vi "Decode data format.vi"(11 "Generic packet":T3) -> (1 "XAM Data Packet":T1, 2 "IDRA Data Packet":T2, 3 "Telemetria.Data format":enum16{"IDRA data", "XAM data"}(ring))   [LabVIEW 2015, in "Acquisition.lvlib"]
uses:
  Acquisition.lvlib
  Generic data packet.ctl
  My Graphs/Gps Map Graph coordinates.ctl
  IDRA Data Packet.ctl
  XAM Data Packet.ctl
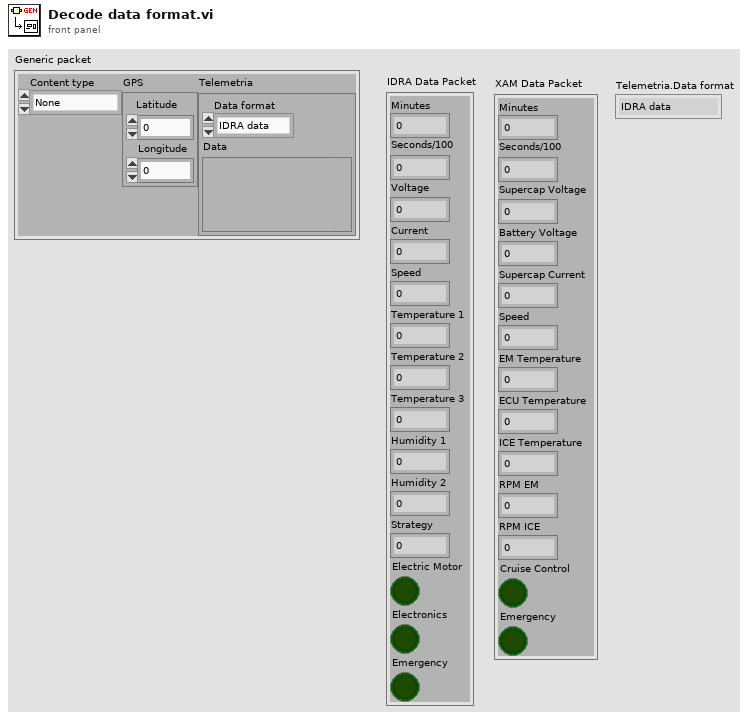
[diagram p1: front panel]
types:
  T1 = typedef "Acquisition.lvlib/XAM Data Packet.ctl" = cluster{"Minutes":u16, "Seconds/100":u16, "Supercap Voltage":sgl, "Battery Voltage":sgl, "Supercap Current":sgl, "Speed":sgl, "EM Temperature":sgl, "ECU Temperature":sgl, "ICE Temperature":sgl, "RPM EM":u16, "RPM ICE":u16, "Cruise Control":bool, "Emergency":bool}
  T2 = typedef "Acquisition.lvlib/IDRA Data Packet.ctl" = cluster{"Minutes":u16, "Seconds/100":u16, "Voltage":sgl, "Current":sgl, "Speed":sgl, "Temperature 1":sgl, "Temperature 2":sgl, "Temperature 3":sgl, "Humidity 1":sgl, "Humidity 2":sgl, "Strategy":u8, "Electric Motor":bool, "Electronics":bool, "Emergency":bool}
  T3 = typedef "Acquisition.lvlib/Generic data packet.ctl" = cluster{"Content type":enum16{"None", "Telemetria", "GPS"}, "GPS":T4, "Telemetria":cluster{"Data format":enum16{"IDRA data", "XAM data"}, "Data":variant}}
  T4 = typedef "Gps Map Graph coordinates.ctl" = cluster{"Latitude":dbl, "Longitude":dbl}
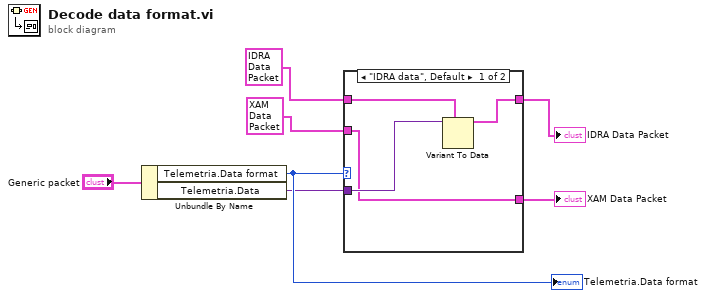
[diagram p0: block diagram]
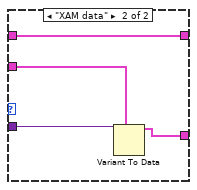
[diagram p2: hidden frame]
diagram:
  n1 = Unbundle By Name("Generic packet") -> ("Telemetria.Data format"=w6:enum16{"IDRA data", "XAM data"}, "Telemetria.Data"=w5:variant)
  "Telemetria.Data format" <- w6
  n2 = case shown="\"IDRA data\", Default" w6 {
    tunnel: w5 -> [w11 w15]
    tunnel: [w8 w14] -> w4
    tunnel: T2 {"Minutes"=0, "Seconds/100"=0, "Voltage"=0.0, "Current"=0.0, "Speed"=0.0, "Temperature 1"=0.0, "Temperature 2"=0.0, "Temperature 3"=0.0, "Humidity 1"=0.0, "Humidity 2"=0.0, "Strategy"=0, "Electric Motor"=FALSE, "Electronics"=FALSE, "Emergency"=FALSE} ("IDRA Data Packet") -> [w10 w12]
    tunnel: T1 {"Minutes"=0, "Seconds/100"=0, "Supercap Voltage"=0.0, "Battery Voltage"=0.0, "Supercap Current"=0.0, "Speed"=0.0, "EM Temperature"=0.0, "ECU Temperature"=0.0, "ICE Temperature"=0.0, "RPM EM"=0, "RPM ICE"=0, "Cruise Control"=FALSE, "Emergency"=FALSE} ("XAM Data Packet") -> [w8 w13]
    tunnel: [w9 w12] -> w1
    frame "IDRA data", Default {
      n3 = Variant To Data(type=w10, Variant=w11) -> (data=w9:T2)  [unwired: 1 in, 1 out]
    }
    frame "XAM data" {
      n4 = Variant To Data(type=w13, Variant=w15) -> (data=w14:T1)  [unwired: 1 in, 1 out]
    }
  }
  "IDRA Data Packet" <- w1
  "XAM Data Packet" <- w4
